vi "Configure Sequencer List Inc Transition.vi"(7 "Inc Transition (Immediate)":i32(ring) items=["Immediate", "Restart Marker", "Waveform Marker 1", "Waveform Marker 2", "Waveform Marker 3", "Waveform Marker 4"], 8 "error in (no error)":errorcluster, 9 "Index (0)":i32, 10 "Instance (1)":i32=1, 11 "VISA resource name":refnum<visa-resource-name>) -> (0 "error out":errorcluster, 3 "VISA resource name out":refnum<visa-resource-name>)   [LabVIEW 2020, in "Rohde&Schwarz CMXP GPRF.lvlib"]
doc: "Defines a condition for the transition to the next list entry, for the sequencer list entry with the selected Index.\n\nAttribute:\nRSCMXPGPRF_ATTR_SEQUENCER_LIST_INC_TRANSITION\n\nRemote-control command:\nSOURce:GPRF:GEN<i>:SEQuencer:LIST:ITRansition"
uses:
  <instrlib>/Rohde&Schwarz CMXP GPRF/Rohde&Schwarz CMXP GPRF.lvlib
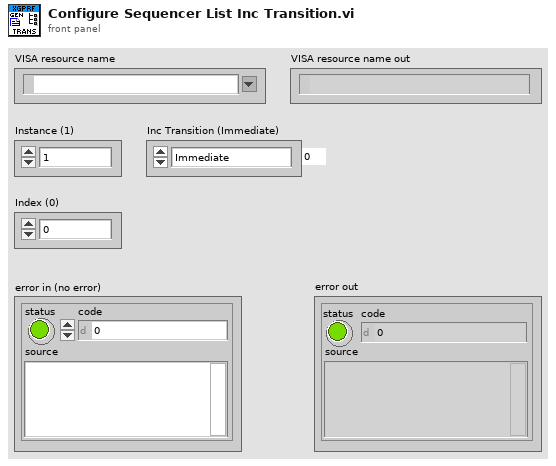
[diagram p1: front panel]
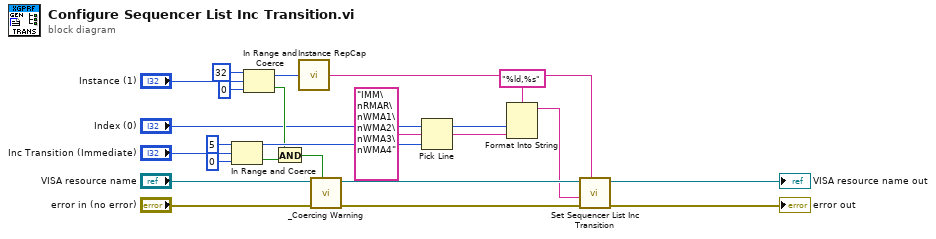
[diagram p0: block diagram]
diagram:
  n1 = In Range and Coerce(upper limit=5, x="Inc Transition (Immediate)", lower limit=0) -> (coerced(x)=w18:i32, In Range?=w12:bool)
  n2 = In Range and Coerce(upper limit=32, x="Instance (1)", lower limit=0) -> (coerced(x)=w10:i32, In Range?=w11:bool)
  n3 = And(x=w11, y=w12) -> (x .and. y?=w13:bool)
  n4 = call <instrlib>:"Instance RepCap.vi"("Instance in"=w10) -> ("Instance out"=w5:string)
  n5 = call <instrlib>:"_Coercing Warning.vi"("In Range?"=w13, "error in (no error)"="error in (no error)", "VISA resource name"="VISA resource name") -> ("error out"=w9:errorcluster, "VISA resource name out"=w8:refnum<visa-resource-name>)  [unwired: 7 in]
  n6 = Pick Line(multi-line string="IMM\nRMAR\nWMA1\nWMA2\nWMA3\nWMA4" ("format string"), line index=w18) -> (output string=w2:string)  [unwired: 1 in]
  n7 = Format Into String(format string="%ld,%s", "Index (0)", w2) -> (resulting string=w1:string)  [unwired: 2 in, 1 out]
  n8 = call "Set Sequencer List Inc Transition"("Repeated Capabilities"=w5, "error in (no error)"=w9, "Sequencer List Inc Transition ()"=w1, "instrument handle"=w8) -> ("error out"=→"error out":errorcluster, "instrument handle out"=→"VISA resource name out":refnum<visa-resource-name>)  [unwired: 6 in]
